vi "getType.vi"(8 "error in (no error)":errorcluster, 11 "IDataRule in":refnum<class "IDataRule.lvclass">) -> (0 "error out":errorcluster, 2 "DataRuleType":T1 items=["daqDataRuleTypeOther ", "daqDataRuleTypeLinear", "daqDataRuleTypeConstant", "daqDataRuleTypeExplicit   "], 3 "IDataRule out":refnum<class "IDataRule.lvclass">)   [LabVIEW 2022 SP3, in "openDAQ.lvlib" / "IBaseObject.lvlib" / "IDataRule.lvlib" / "IDataRule.lvclass"]
uses:
  <instrlib>/openDAQ/Public/Classes/IDataRule/IDataRule.lvclass
  <instrlib>/openDAQ/Public/Classes/IDataRule/IDataRule.lvclass/IDataRule.ctl
  <instrlib>/openDAQ/Binaries/Windows/x86/copendaq32.dll
  <instrlib>/openDAQ/Public/Classes/IDataRule/TypeDef/DataRuleType.ctl
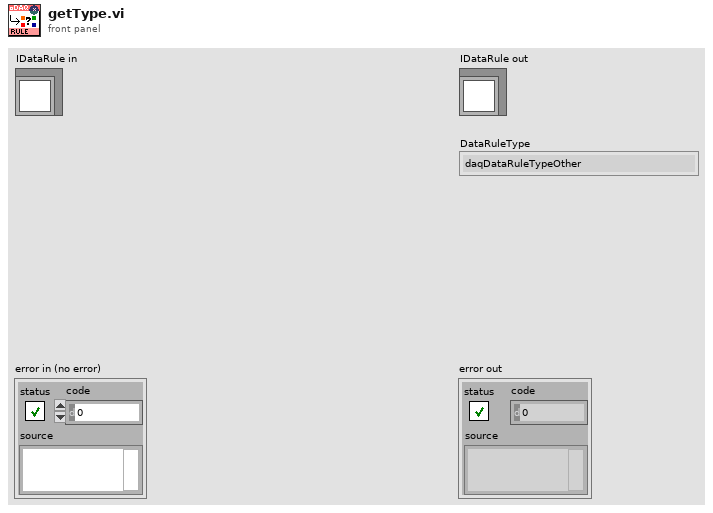
[diagram p1: front panel]
types:
  T1 = typedef "openDAQ.lvlib/IBaseObject.lvlib/IDataRule.lvlib/IDataRule.lvclass/DataRuleType.ctl" = u16
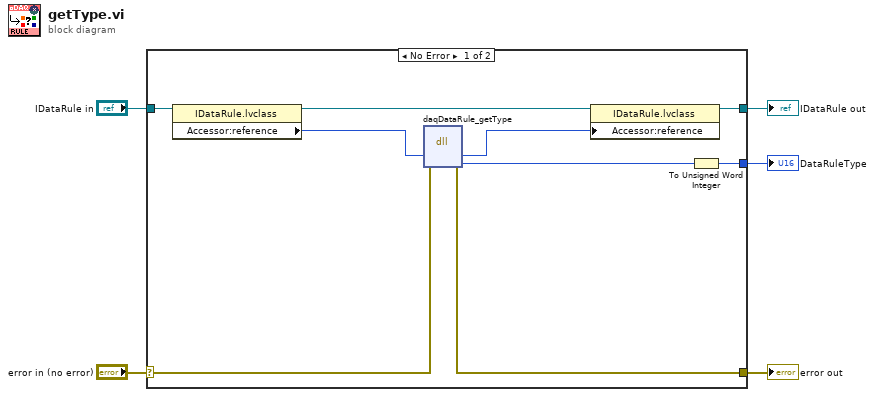
[diagram p0: block diagram]
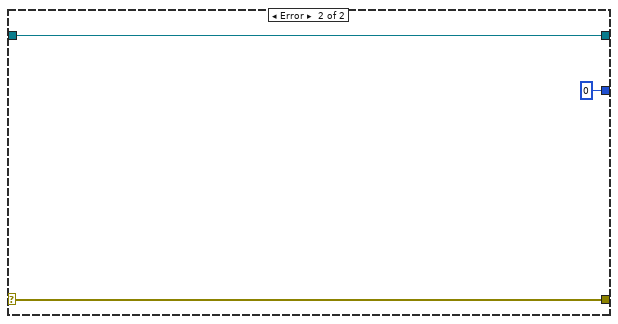
[diagram p2: hidden frame]
diagram:
  n1 = case shown="No Error" "error in (no error)" {
    selector: "error in (no error)" -> [w13 w17]
    tunnel: [w12 w17] -> w4
    tunnel: [w6 w16] -> w2
    tunnel: "IDataRule in" -> [w14 w16]
    tunnel: [w9 u16 0] -> w1
    frame No Error {
      n2 = property class="IDataRule.lvclass"(reference=w14) -> (reference out=w7:refnum<class "IDataRule.lvclass">, "Accessor:reference"=w11:i64)  [unwired: 1 in, 1 out]
      n3 = dll-call lib="C:/Program Files (x86)/National Instruments/LabVIEW 2022/instr.lib/openDAQ/Binaries/Windows/x86/copendaq*.*" fn="daqDataRule_getType"(error in=w13, "dataRule"=w11) -> (error out=w12:errorcluster, "dataRule"=w8:i64, "dataRuleType"=w10:i64)  [unwired: 4 in, 1 out]
      n4 = property class="IDataRule.lvclass"(reference=w7, "Accessor:reference"=w8) -> (reference out=w6:refnum<class "IDataRule.lvclass">)  [unwired: 1 in, 1 out]
      n5 = To Unsigned Word Integer(number=w10) -> (unsigned 16bit integer=w9:u16)
    }
    frame Error {
    }
  }
  "error out" <- w4
  "IDataRule out" <- w2
  "DataRuleType" <- w1
